vi "GetCurrent.vi"(8 "Error In":errorcluster, 11 "reference in":refnum<class "BreakfastMenuEnum.lvclass">) -> (0 "Error Out":errorcluster, 2 "Current":refnum<class "Menu.lvclass">, 3 "reference out":refnum<class "BreakfastMenuEnum.lvclass">)   [LabVIEW 2020, in "BreakfastMenuEnum.lvclass"]
uses:
  BreakfastMenuEnum.lvclass
  Menu_class/Menu.lvclass
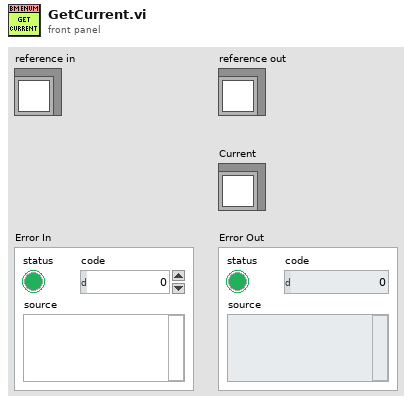
[diagram p1: front panel]
types:
  T1 = typedef "BreakfastMenuEnum.lvclass/ObjectAttributes.ctl" = cluster{"_items":variant[], "_position":i32, "IEnumerator.Current":refnum<class>, "Current":refnum<class "Menu.lvclass">}
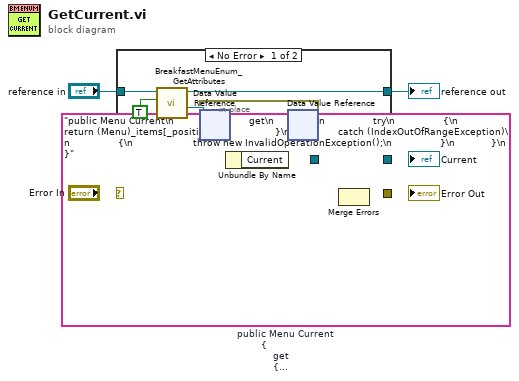
[diagram p0: block diagram]
diagram:
  (unwired) "public Menu Current\n        {\n            get\n            {\n                try\n                {\n                    return (Menu)_items[_position];\n                }\n                catch (IndexOutOfRangeException)\n                {\n                    throw new InvalidOperationException();\n                }\n            }\n        }"  # public Menu Current         {             get             {                 try                 {                     return (Menu)_items[_position];                 }                 catch (IndexOutOfRangeException)                 {                     throw new InvalidOperationException();                 }             }         }
  n1 = case shown="No Error" "Error In" {
    selector: "Error In" -> [w14 w18]
    tunnel: [w12 w18] -> w4
    tunnel: [w9 w17] -> w2
    tunnel: "reference in" -> [w10 w17]
    tunnel: [w6 _] -> w1
    frame No Error {
      n2 = call "BreakfastMenuEnum_GetAttributes.vi"("error in (no error)"=w14, "OnlyGetDvrReference(False)"=TRUE, "reference in"=w10) -> ("error out"=w13:errorcluster, "DataRef"=w7:refnum<data-value>, "reference out"=w9:refnum<class "BreakfastMenuEnum.lvclass">)  [unwired: 5 in, 1 out]
      n3 = in-place {
        in-place-border: [w16] -> w6
        n4 = in-place-dvr #1(w7) -> (w15:T1)  [unwired: 1 out]
        n5 = Unbundle By Name(w15) -> ("Current"=w16:refnum<class "Menu.lvclass">)
        n6 = in-place-dvr #1(w15) -> (w11:errorcluster)  [unwired: 1 out]
      }
      n7 = Merge Errors(w13, w11) -> (w12:errorcluster)
    }
    frame Error {
    }
  }
  "Error Out" <- w4
  "reference out" <- w2
  "Current" <- w1
